vi "getTimeStamp.vi"() -> (0 "Time Stamp":timestamp)   [LabVIEW 2015]
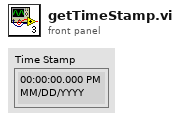
[diagram p1: front panel]
types:
  T1 = cluster{dbl, i32, i32, i32, i32, i32, i32, i32, i32, i32}
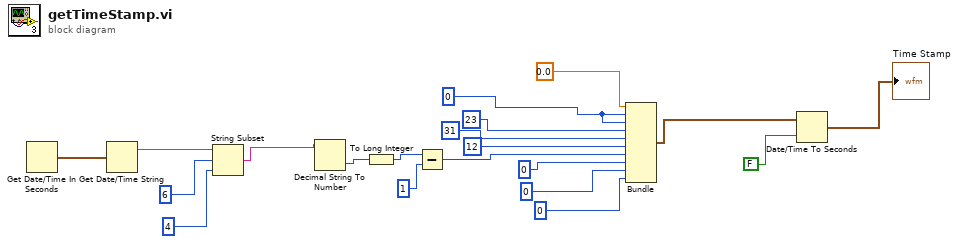
[diagram p0: block diagram]
diagram:
  w5 = 0
  (unwired) 6
  n1 = Get Date/Time In Seconds() -> (seconds since 1Jan1904=w20:timestamp)
  n2 = Get Date/Time String(seconds (now)=w20) -> (date string=w19:string)  [unwired: 2 in, 1 out]
  n3 = String Subset(string=w19, offset (0)=6, length (rest)=4) -> (substring=w10:string)
  n4 = Decimal String To Number(string=w10) -> (number=w9:i32)  [unwired: 2 in, 1 out]
  n5 = To Long Integer(number=w9) -> (32bit integer=w3:i32)
  n6 = Subtract(x=w3, y=1) -> (x-y=w1:i32)
  n7 = Bundle(0.0, w5, w5, 23, 31, 12, w1, 0, 0, 0) -> (w6:T1)  [unwired: 1 in]
  n8 = Date/Time To Seconds(1:FALSE, 2:w6) -> (0:→"Time Stamp":timestamp)
